vi "打开工作簿集.vi"(8 "错误输入（无错误）":errorcluster) -> (0 "错误输出":errorcluster, 2 "工作簿集":refnum<k7>, 3 "excel.application输出":refnum<k7>)   [LabVIEW 2013, in "excel处理.lvlib"]
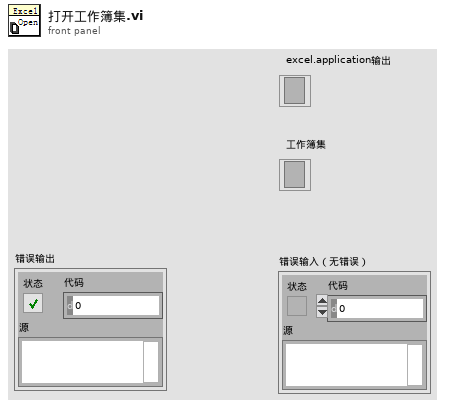
[diagram p1: front panel]
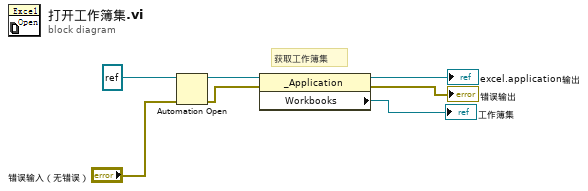
[diagram p0: block diagram]
diagram:
  # "获取工作簿集"
  n1 = Automation Open(error in (no error)="错误输入（无错误）", Automation Refnum=refnum<k7> refnum ("Excel._Application")) -> (Automation Refnum=w6:refnum<k7>, error out=w4:errorcluster)  [unwired: 2 in]
  n2 = property on="属性节点" class="_Application"(reference=w6, error in=w4) -> (reference out=→"excel.application输出":refnum<k7>, error out=→"错误输出":errorcluster, "Workbooks"=→"工作簿集":refnum<k7>)
